vi "WT500 Misc Cmd.vi"(8 "error in":errorcluster, 10 "Write Data":string, 11 "VISA resource name":refnum<visa-resource-name>) -> (0 "error out":errorcluster, 2 "Read Data":string, 3 "VISA resource name out":refnum<visa-resource-name>)   [LabVIEW 2016]
panel:
  out "Data Length":i32
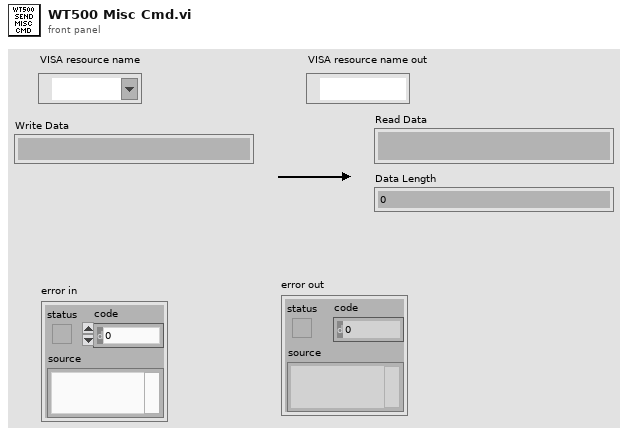
[diagram p1: front panel]
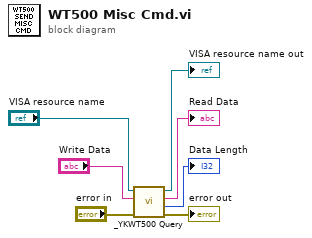
[diagram p0: block diagram]
diagram:
  n1 = call "_YKWT500 Query.vi"("error in (no error)"="error in", "Write Data"="Write Data", "VISA resource name"="VISA resource name") -> ("error out"=→"error out":errorcluster, "Data Length"=→"Data Length":i32, "Read Data"=→"Read Data":string, "VISA resource name out"=→"VISA resource name out":refnum<visa-resource-name>)  [unwired: 5 in]
